vi "Test Barista Sends Pick Up Callback.vi"(8 "error in (no error)":errorcluster, 11 "Barista Test in":refnum<class "Barista Test.lvclass">) -> (0 "error out":errorcluster, 3 "Barista Test out":refnum<class "Barista Test.lvclass">)   [LabVIEW 2020, in "Barista Test.lvclass"]
uses:
  Barista Test.lvclass
  C:/Program Files (x86)/National Instruments/LabVIEW 2020/vi.lib/Asteme/LUnit/Test Case.lvclass
  Barista/Barista.lvclass
  C:/Program Files (x86)/National Instruments/LabVIEW 2020/vi.lib/Asteme/Triarc Framework/Process/Process.lvclass
  Support/Beverages/Beverage/Beverage.lvclass
  Mock Pick Up Order/Mock Pick Up Order.lvclass
  C:/Users/anton/Documents/GitHub/Triarc-Examples/Coffee Shop/Pick Up Order/Pick Up Order.lvclass
  Support/Beverages/TypeDefs/Drink Type.ctl
  Support/Beverages/TypeDefs/Options.ctl
  Support/Beverages/Beverage/Beverage.lvclass/Beverage.ctl
  <vilib>/Asteme/Triarc Framework/Process/Process.lvclass/Process.ctl
  <vilib>/Asteme/LUnit/Test Case.lvclass/Test Case.ctl
  <vilib>/Asteme/LUnit/LUnit Assertion Result.lvclass/LUnit Assertion Result.ctl
  Support/Beverages/Beverage/Write Drink Type.vi
  Support/Beverages/Beverage/Write Options.vi
  <vilib>/Asteme/Triarc Framework/Process/Private/SubVIs/Wait for finish.vi
  <vilib>/Asteme/Triarc Framework/Process/Protected/Messaging/Enqueue Message.vi
  <vilib>/Asteme/Triarc Framework/Process/Private/SubVIs/Set Lifecycle State.vi
  <vilib>/Asteme/Triarc Framework/Process/Public/Lifecycle/Get Lifecycle State.vi
  <vilib>/Asteme/LUnit/Palette/Pass.vi
  <vilib>/Asteme/LUnit/Palette/Fail.vi
  <vilib>/Asteme/LUnit/Variant to string.vi
  <vilib>/Asteme/LUnit/Set Assertion Type.vi
  <vilib>/Utility/error.llb/Clear Errors.vi
  <vilib>/Asteme/LUnit/Add test result.vi
  <vilib>/Asteme/LUnit/LUnit Write Passed.vi
  <vilib>/Asteme/LUnit/LUnit Get Test Case.vi
  <vilib>/Asteme/LUnit/Assertion Result/LUnit Get Test Name.vi
  <vilib>/Asteme/LUnit/LUnit Write Message.vi
  <vilib>/Asteme/LUnit/LUnit Write Description.vi
  <vilib>/Asteme/LUnit/LUnit Write Assertion Type.vi
  <vilib>/Asteme/LUnit/Read Test Case Name.vi
  <vilib>/Utility/error.llb/Error Cluster From Error Code.vi
  <vilib>/Utility/Data Type/Get Type Information.vi
  <vilib>/Utility/LVClass/Get LV Class Name.vi
  <vilib>/Asteme/LUnit/LUnit Assertion Result.lvclass
  <vilib>/Asteme/Triarc Framework/Process/Process.lvclass
  Support/Order Item/Order Item.lvclass
  <vilib>/Asteme/LUnit/Test Case.lvclass
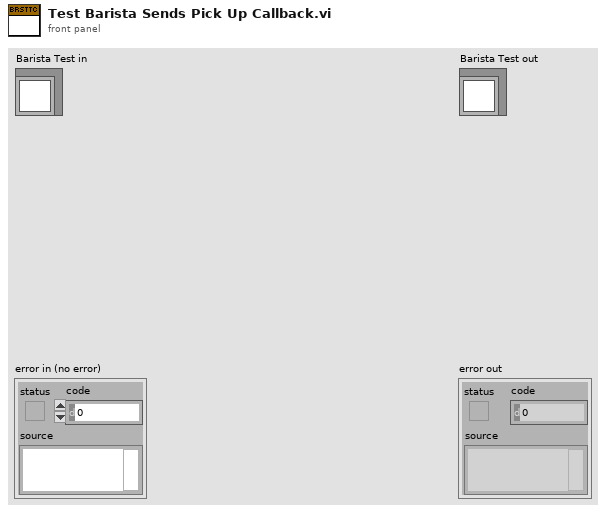
[diagram p1: front panel]
types:
  T1 = typedef "Beverage.lvclass/Options.ctl" = enum16{"<None>", "Milk", "Mocha", "Soy", "Whip"}
  T2 = typedef "Beverage.lvclass/Drink Type.ctl" = enum16{"Dark Roast", "Decaf", "Espresso", "House Blend"}
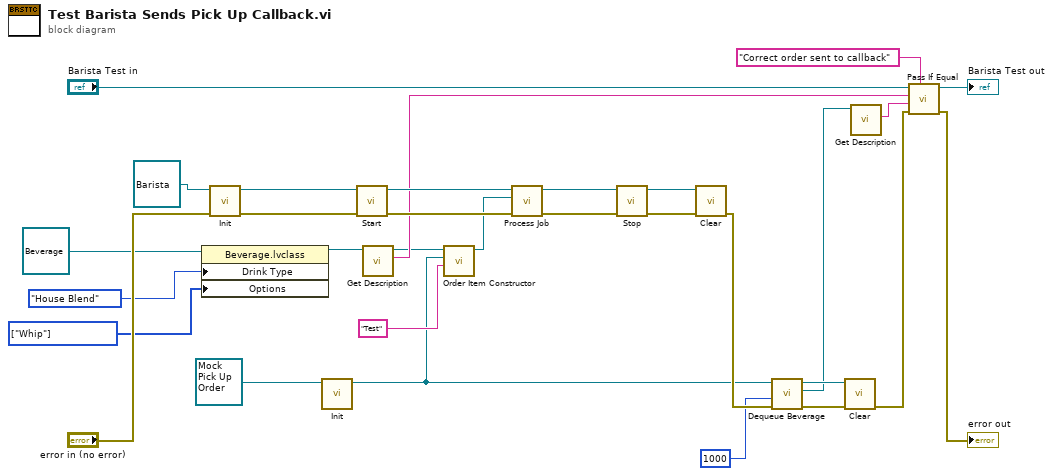
[diagram p0: block diagram]
diagram:
  w3 = T1[] [enum."Whip"] items=["<None>", "Milk", "Mocha", "Soy", "Whip"] ("Options")
  n1 = property class="Beverage.lvclass"(reference=refnum<class "Beverage.lvclass"> refnum ("Beverage"), "Drink Type"=Drink_Type."House Blend", "Options"=w3) -> (reference out=w2:refnum<class "Beverage.lvclass">)  [unwired: 1 in, 1 out]
  n2 = call-dynamic "Init.vi"("error in (no error)"="error in (no error)", "View In"=refnum<class "Barista.lvclass"> refnum ("Barista.lvclass")) -> ("error out"=w28:errorcluster, "View Out"=w24:refnum<class "Barista.lvclass">)  [unwired: 8 in]
  n3 = call-dynamic "Init.vi"("Mock Worker In"=refnum<class "Mock Pick Up Order.lvclass"> refnum ("Mock Pick Up Order.lvclass")) -> ("Mock Worker Out"=w6:refnum<class "Mock Pick Up Order.lvclass">)  [unwired: 9 in, 1 out]
  n4 = call <vilib>:"Start.vi"("error in (no error)"=w28, "Process In"=w24) -> ("error out"=w30:errorcluster, "Process Out"=w23:refnum<class "Barista.lvclass">)  [unwired: 8 in]
  n5 = call "Get Description.vi"("Beverage in"=w2) -> ("Description"=w14:string, "Beverage out"=w1:refnum<class "Beverage.lvclass">)  [unwired: 8 in, 1 out]
  n6 = call "Order Item Constructor.vi"("Cust Name"="Test", "Pick Up Order.lvclass"=w6, "Beverage"=w1) -> ("Order Item"=w26:refnum<class "Order Item.lvclass">)  [unwired: 7 in, 1 out]
  n7 = call-dynamic "Process Job.vi"("error in (no error)"=w30, "Job"=w26, "Worker In"=w23) -> ("error out"=w20:errorcluster, "Worker Out"=w22:refnum<class "Barista.lvclass">)  [unwired: 7 in]
  n8 = call <vilib>:"Stop.vi"("error in (no error)"=w20, "Process In"=w22) -> ("error out"=w29:errorcluster, "Process Out"=w21:refnum<class "Barista.lvclass">)  [unwired: 7 in, 1 out]
  n9 = call-dynamic "Clear.vi"("error in (no error)"=w29, "View In"=w21) -> ("error out"=w18:errorcluster)  [unwired: 9 in]
  n10 = call "Dequeue Beverage.vi"("error in (no error)"=w18, "timeout in ms (-1)"=1000, "Mock Worker in"=w6) -> ("error out"=w13:errorcluster, "Beverage"=w10:refnum<class "Beverage.lvclass">, "Mock Worker out"=w12:refnum<class "Mock Pick Up Order.lvclass">)  [unwired: 5 in, 1 out]
  n11 = call-dynamic "Clear.vi"("error in (no error)"=w13, "Mock Worker In"=w12) -> ("error out"=w9:errorcluster)  [unwired: 9 in]
  n12 = call "Get Description.vi"("Beverage in"=w10) -> ("Description"=w11:string)  [unwired: 8 in, 2 out]
  n13 = call <vilib>:"Pass If Equal.vi"("Description"="Correct order sent to callback", "error in (no error)"=w9, "Actual"=w11, "Expected"=w14, "Test Case In"="Barista Test in") -> ("error out"=→"error out":errorcluster, "Test Case Out"=→"Barista Test out":refnum<class "Barista Test.lvclass">)  [unwired: 5 in]
